vi "Clear Hardware.vi"(2 "error in (no error)":errorcluster, 3 "Novatech in":refnum<class "Novatech.lvclass">) -> (0 "error out":errorcluster, 1 "Novatech out":refnum<class "Novatech.lvclass">)   [LabVIEW 2013, in "Novatech.lvclass"]
uses:
  Novatech.lvclass
  Novatech.lvclass/Novatech.ctl
  Novatech 409A.lvlib
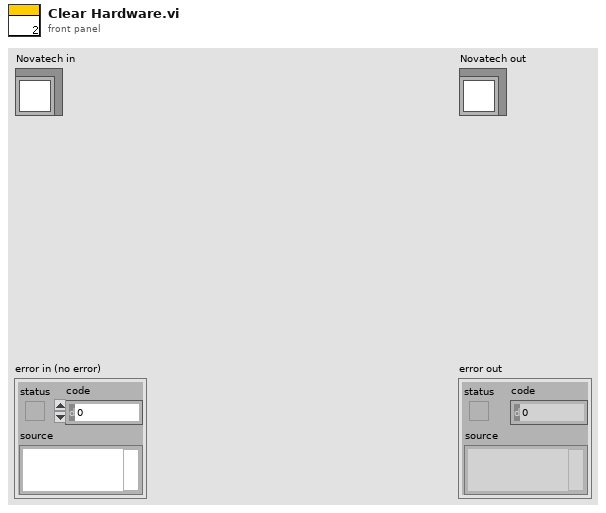
[diagram p1: front panel]
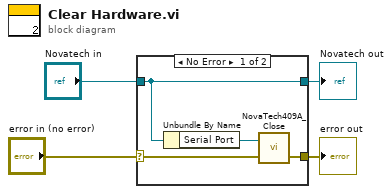
[diagram p0: block diagram]
diagram:
  n1 = case shown="No Error" "error in (no error)" {
    selector: "error in (no error)" -> [w8 w10]
    tunnel: "Novatech in" -> [w7 w9]
    tunnel: [w7 w9] -> w2
    tunnel: [w6 w10] -> w1
    frame No Error {
      n2 = Unbundle By Name(w7) -> ("Serial Port"=w5:refnum<visa-resource-name>)
      n3 = call "NovaTech409A_Close.vi"("error in (no error)"=w8, "VISA resource name"=w5) -> ("error out"=w6:errorcluster)  [unwired: 1 out]
    }
    frame Error {
    }
  }
  "error out" <- w1
  "Novatech out" <- w2
